vi "Update Position to Globals.vi"(8 "Error In":errorcluster) -> (0 "Error Out":errorcluster)   [LabVIEW 2012]
uses:
  <vilib>/DAQmx/write.llb/DAQmx Write (Analog 1D DBL NChan 1Samp).vi
  Channels.vi
  <vilib>/DAQmx/create/channels.llb/DAQmx Create Channel (AO-Voltage-Basic).vi
  Global Vars.vi
  <vilib>/DAQmx/miscellaneous.llb/DAQmx Fill In Error Info.vi
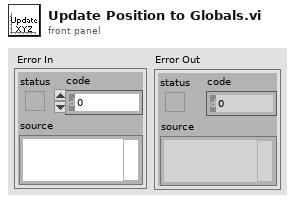
[diagram p1: front panel]
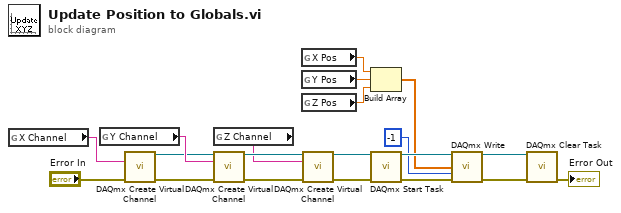
[diagram p0: block diagram]
diagram:
  n1 = global read "Channels.vi" "X Channel"() -> (w15:tag)
  n2 = global read "Channels.vi" "Y Channel"() -> (w10:tag)
  n3 = call-poly <vilib>:"DAQmx Create Virtual Channel.vi"("physical channels"=w15, "error in"="Error In") -> ("task out"=w9:refnum<k21>, "error out"=w8:errorcluster)  [unwired: 12 in]
  n4 = global read "Channels.vi" "Z Channel"() -> (w1:tag)
  n5 = call-poly <vilib>:"DAQmx Create Virtual Channel.vi"("task in"=w9, "physical channels"=w10, "error in"=w8) -> ("task out"=w3:refnum<k21>, "error out"=w2:errorcluster)  [unwired: 11 in]
  n6 = global read "Global Vars.vi" "X Pos"() -> (w13:dbl)
  n7 = global read "Global Vars.vi" "Y Pos"() -> (w12:dbl)
  n8 = global read "Global Vars.vi" "Z Pos"() -> (w6:dbl)
  n9 = call-poly <vilib>:"DAQmx Create Virtual Channel.vi"("task in"=w3, "physical channels"=w1, "error in"=w2) -> ("task out"=w5:refnum<k21>, "error out"=w4:errorcluster)  [unwired: 11 in]
  n10 = Build Array(w13, w12, w6) -> (w7:dbl[])
  n11 = call <vilib>:"DAQmx Start Task.vi"("task/channels in"=w5, "error in"=w4) -> ("task out"=w20:refnum<k21>, "error out"=w18:errorcluster)  [unwired: 12 in]
  n12 = call-poly <vilib>:"DAQmx Write.vi"("task/channels in"=w20, "data"=w7, "timeout"=-1, "error in"=w18) -> ("task out"=w19:refnum<k21>, "error out"=w17:errorcluster)  [unwired: 9 in, 1 out]
  n13 = call <vilib>:"DAQmx Clear Task.vi"("task in"=w19, "error in"=w17) -> ("error out"=→"Error Out":errorcluster)  [unwired: 13 in]
